vi "Motor Power.vi"(9 "Motor":i16, 11 "data":waveform(dbl)[](array[waveform])) -> (1 "Power":waveform(dbl), 2 "Phase Current":waveform(dbl)(graph), 3 "Phase to Phase Voltage":waveform(dbl)(graph), 4 "Voltage 2":waveform(dbl))   [LabVIEW 2011]
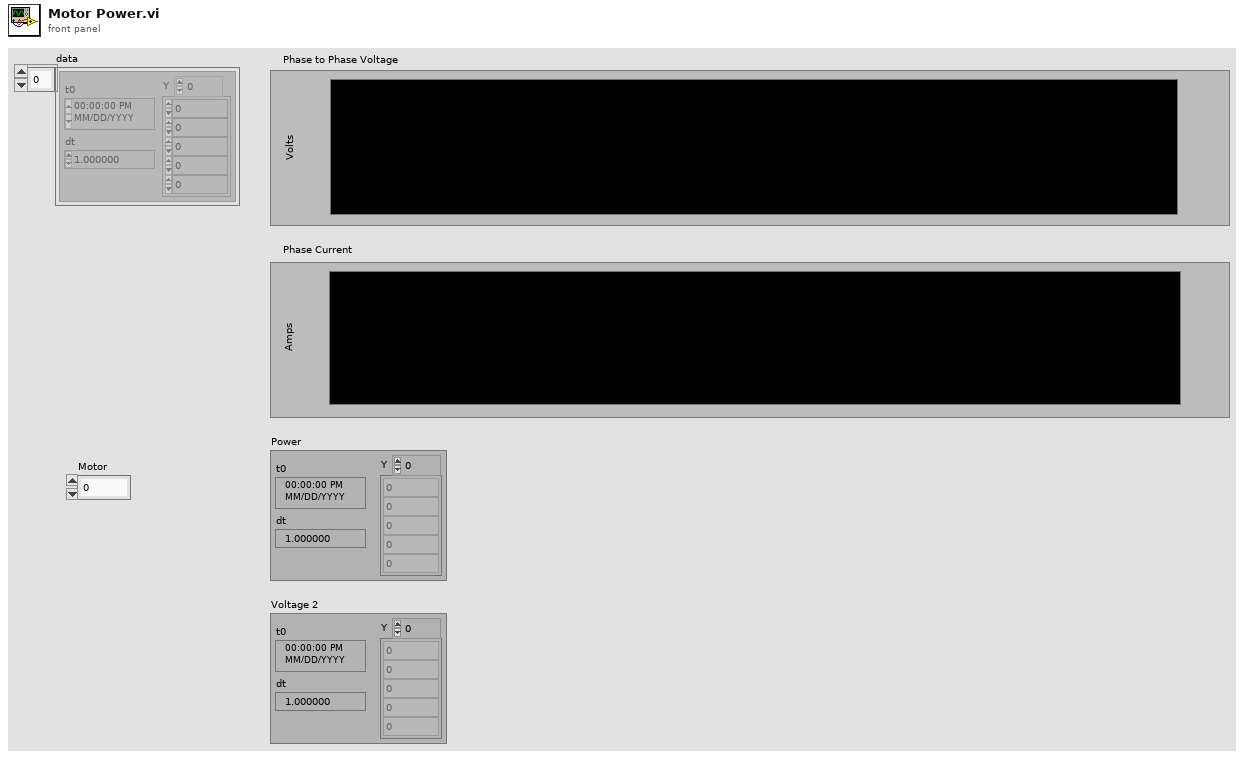
[diagram p1: front panel]
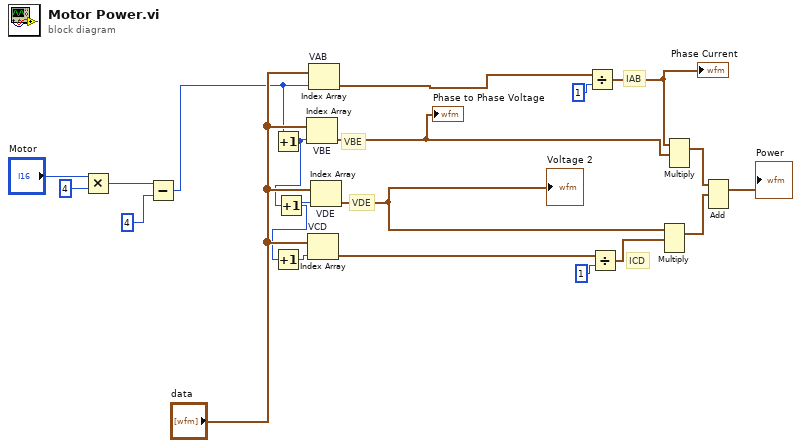
[diagram p0: block diagram]
diagram:
  # "IAB"
  # "VBE"
  # "ICD"
  # "VDE"
  n1 = Multiply(x="Motor", y=i16 4) -> (x*y=w2:i16)
  n2 = Subtract(x=w2, y=i16 4) -> (x-y=w3:i16)
  n3 = Increment(x=w3) -> (x+1=w4:i16)
  n4 = Increment(x=w4) -> (x+1=w5:i16)
  n5 = Increment(x=w5) -> (x+1=w6:i16)
  n6 = Index Array "VBE"(array="data", index=w4) -> (element=w18:waveform(dbl))
  "Phase to Phase Voltage" <- w18
  n7 = Index Array "VCD"(array="data", index=w6) -> (element=w19:waveform(dbl))
  n8 = Index Array "VAB"(array="data", index=w3) -> (element=w17:waveform(dbl))
  n9 = Index Array "VDE"(array="data", index=w5) -> (element=w10:waveform(dbl))
  "Voltage 2" <- w10
  n10 = Divide(x=w17, y=1) -> (x/y=w16:waveform(dbl))
  "Phase Current" <- w16
  n11 = Divide(x=w19, y=1) -> (x/y=w9:waveform(dbl))
  n12 = Multiply(1:w9, 2:w10) -> (0:w13:waveform(dbl))  [unwired: 1 in, 1 out]
  n13 = Multiply(1:w18, 2:w16) -> (0:w11:waveform(dbl))  [unwired: 1 in, 1 out]
  n14 = Add(1:w13, 2:w11) -> (0:→"Power":waveform(dbl))  [unwired: 1 in, 1 out]
